vi "Read.vi"(7 "Read Type":T1, 8 "error in (no error)":errorcluster, 11 "NetworkStreamReader in":refnum<class "NetworkStreamReader.lvclass">) -> (0 "error out":errorcluster, 1 "New element?":bool, 2 "element":variant, 3 "NetworkStreamReader out":refnum<class "NetworkStreamReader.lvclass">, 4 "Time Stamp":timestamp)   [LabVIEW 2011, in "NetworkStreamReader.lvclass"]
doc: "Returns the requested value (either the next element available in the buffer or the most recent element). If there are no elements available in the queue, this VI will return the last valid value it returned."
uses:
  NetworkStreamReader.lvclass
  readType.ctl
  NetworkStreamReader.lvclass/NetworkStreamReader.ctl
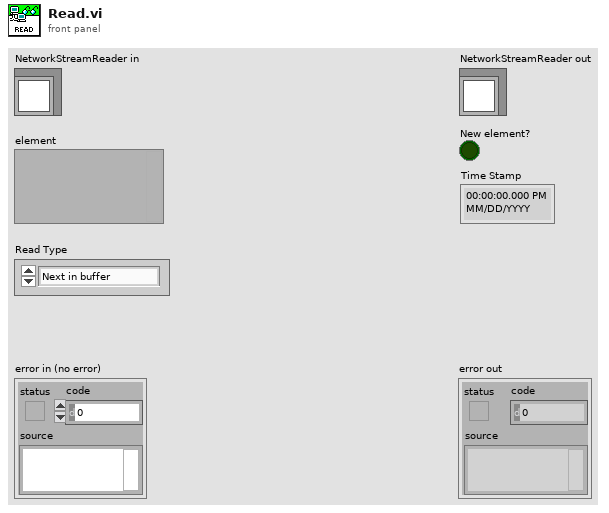
[diagram p1: front panel]
types:
  T1 = typedef "NetworkStreamReader.lvclass/readType.ctl" = enum16{"Next in buffer", "Most current"}
  T2 = typedef "message.ctl" = cluster{"Data":variant, "Time since start (s)":dbl}
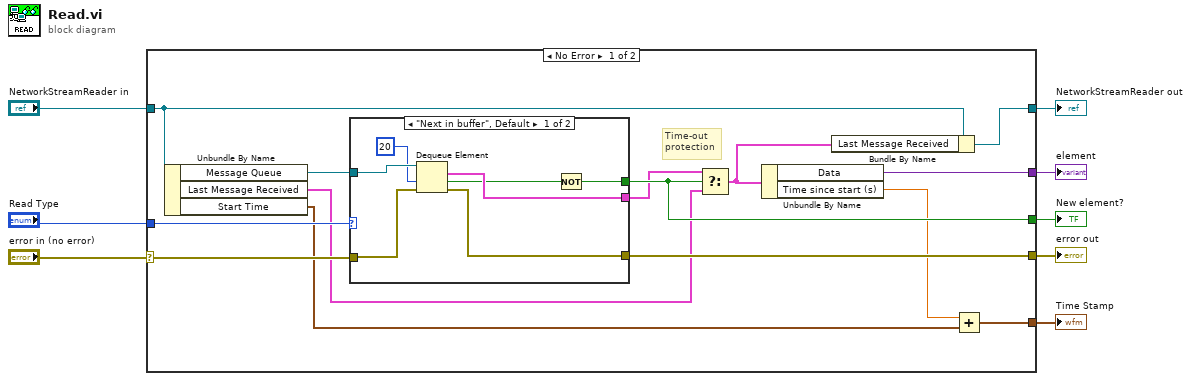
[diagram p0: block diagram]
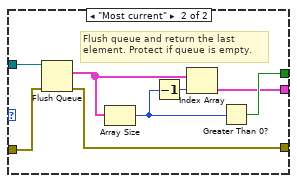
[diagram p2: hidden frame]
diagram:
  n1 = case shown="No Error" "error in (no error)" {
    selector: "error in (no error)" -> [w20 w39]
    tunnel: [w21 w39] -> w7
    tunnel: [w17 w38] -> w6
    tunnel: "NetworkStreamReader in" -> [w18 w38]
    tunnel: [w12 _] -> w5
    tunnel: "Read Type" -> [w19 _]
    tunnel: [w16 _] -> w2
    tunnel: [w14 _] -> w1
    frame No Error {
      # "Time-out \nprotection"
      n2 = Unbundle By Name(w18) -> ("Message Queue"=w22:refnum<queue>, "Last Message Received"=w9:T2, "Start Time"=w15:timestamp)
      n3 = case shown="\"Next in buffer\", Default" w19 {
        tunnel: w22 -> [w29 w37]
        tunnel: [w26 w34] -> w21
        tunnel: w20 -> [w27 w36]
        tunnel: [w24 w35] -> w16
        tunnel: [w25 w30] -> w10
        frame "Next in buffer", Default {
          n4 = Dequeue Element(queue=w29, timeout in ms (-1)=20, error in (no error)=w27) -> (element=w25:T2, timed out?=w23:bool, error out=w26:errorcluster)  [unwired: 1 out]
          n5 = Not(x=w23) -> (.not. x?=w24:bool)
        }
        frame "Most current" {
          # "Flush queue and return the last\nelement. Protect if queue is empty."
          n6 = Flush Queue(queue=w37, error in (no error)=w36) -> (remaining elements=w32:T2[], error out=w34:errorcluster)  [unwired: 1 out]
          n7 = Array Size(array=w32) -> (size(s)=w33:i32)
          n8 = Decrement(x=w33) -> (x-1=w31:i32)
          n9 = Index Array(array=w32, index=w31) -> (element=w30:T2)
          n10 = Greater Than 0?(x=w33) -> (x > 0?=w35:bool)
        }
      }
      n11 = Select(t=w10, s=w16, f=w9) -> (s? t:f=w13:T2)
      n12 = Unbundle By Name(w13) -> ("Data"=w12:variant, "Time since start (s)"=w11:dbl)
      n13 = Bundle By Name(cluster=w18, "Last Message Received"=w13) -> (w17:refnum<class "NetworkStreamReader.lvclass">)
      n14 = Add(x=w11, y=w15) -> (x+y=w14:timestamp)
    }
    frame Error {
    }
  }
  "error out" <- w7
  "NetworkStreamReader out" <- w6
  "element" <- w5
  "New element?" <- w2
  "Time Stamp" <- w1
